vi "Initialise Spectrum Queue.vi"(8 "error in (no error)":errorcluster) -> (0 "error out":errorcluster)   [LabVIEW 2016]
doc: "Initialise the Spectrum queue"
uses:
  Utilities/Application Globals.vi
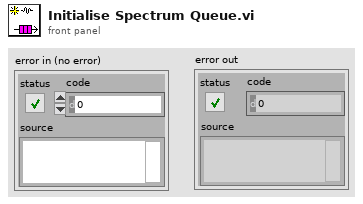
[diagram p1: front panel]
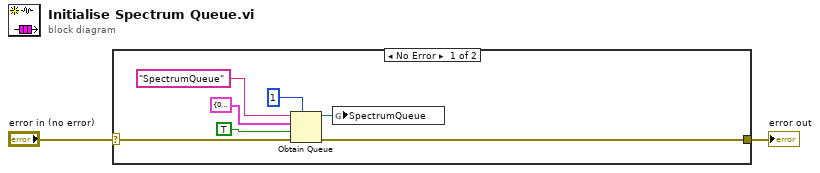
[diagram p0: block diagram]
diagram:
  n1 = case shown="No Error" "error in (no error)" {
    selector: "error in (no error)" -> [w4 w10]
    tunnel: [w3 w10] -> w1
    frame No Error {
      n2 = Obtain Queue(max queue size (-1, unlimited)=1, name (unnamed)="SpectrumQueue", element data type=cluster{"f0":dbl, "df":dbl, "magnitude":dbl[]} {"f0"=0.0, "df"=0.0, "magnitude"=[]} ("output cluster"), create if not found? (T)=TRUE, error in (no error)=w4) -> (queue out=w9:refnum<queue>, error out=w3:errorcluster)  [unwired: 1 out]
      n3 = global write "Application Globals.vi" "SpectrumQueue"(w9) -> ()
    }
    frame Error {
    }
  }
  "error out" <- w1
